vi "Select Items in Listbox_UI.vi"(8 "error in (no error)":errorcluster, 10 "Coords":T5, 11 "Input ListBox Cluster":T1) -> (0 "error out":errorcluster, 3 "ListBox Cluster out":T1)   [LabVIEW 2015, in "ZenGage v3.0 UI.lvclass"]
doc: "This VI checks for selected and unselected measurements."
uses:
  ZenGage v3.0 UI.lvclass
  <vilib>/Utility/miscctls.llb/LVPositionTypeDef.ctl
  Type Definitions/Edit tolerance settings/Edit Tolerance Input.ctl
  Type Definitions/Edit tolerance settings/ETL controls.ctl
  Type Definitions/Edit tolerance settings/Rack Selection.ctl
  <vilib>/Utility/miscctls.llb/LVPoint32TypeDef.ctl
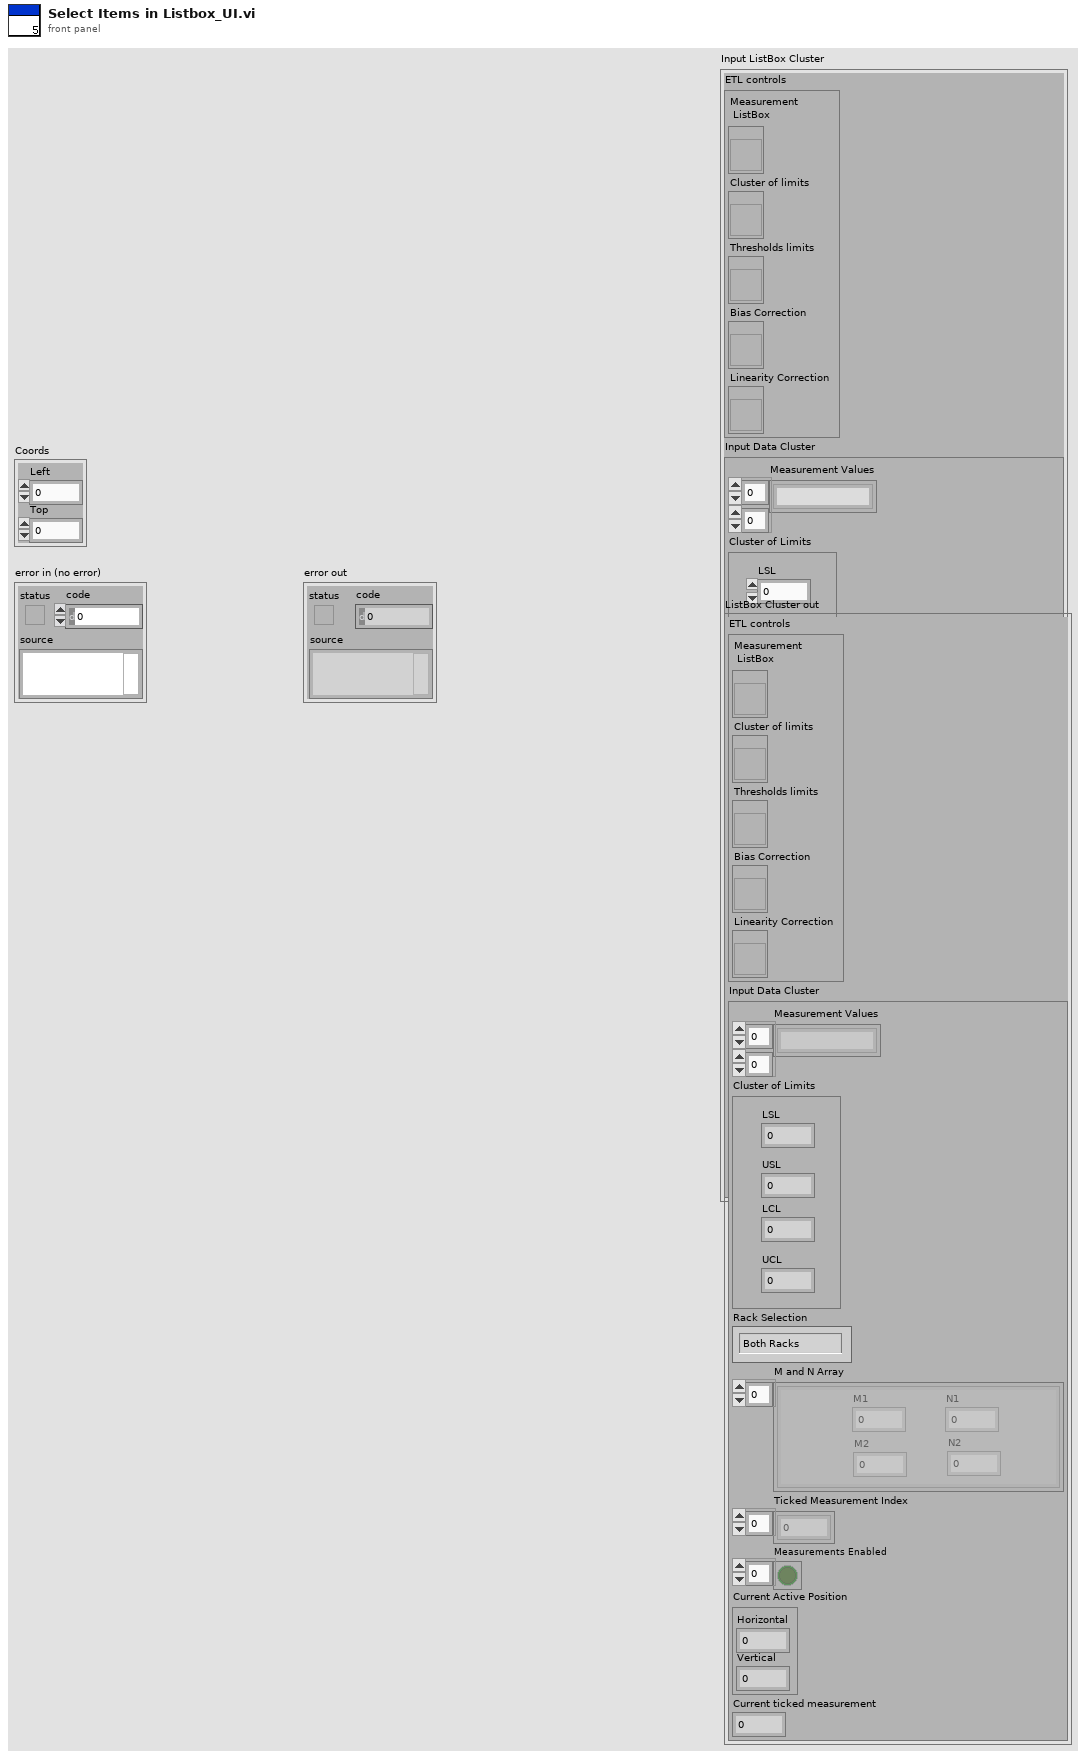
[diagram p1: front panel]
types:
  T1 = typedef "ZenGage v3.0 UI.lvclass/Edit Tolerance Input.ctl" = cluster{"ETL controls":T2, "Input Data Cluster":cluster{"Measurement Values":string[][], "Cluster of Limits":cluster{"LSL":dbl, "USL":dbl, "LCL":dbl, "UCL":dbl}, "Rack Selection":T3, "M and N Array":cluster{"M1":u64, "M2":u64, "N1":u64, "N2":u64}[], "Ticked Measurement Index":u32[], "Measurements Enabled":bool[], "Current Active Position":T4, "Current ticked measurement":dbl}}
  T2 = typedef "ETL controls.ctl" = cluster{"Measurement\n ListBox":refnum<vi>, "Cluster of limits":refnum<vi>, "Thresholds limits":refnum<vi>, "Bias Correction":refnum<vi>, "Linearity Correction":refnum<vi>}
  T3 = typedef "ZenGage v3.0 UI.lvclass/Rack Selection.ctl" = enum16{"Both Racks", "Rack 2", "Rack 1"}
  T4 = typedef "LVPoint32TypeDef.ctl" = cluster{"Horizontal":i32, "Vertical":i32}
  T5 = typedef "LVPositionTypeDef.ctl" = cluster{"Left":i32, "Top":i32}
  T6 = typedef "LVRowAndColumnTypeDef.ctl" = cluster{"Row":i32, "Column":i32}
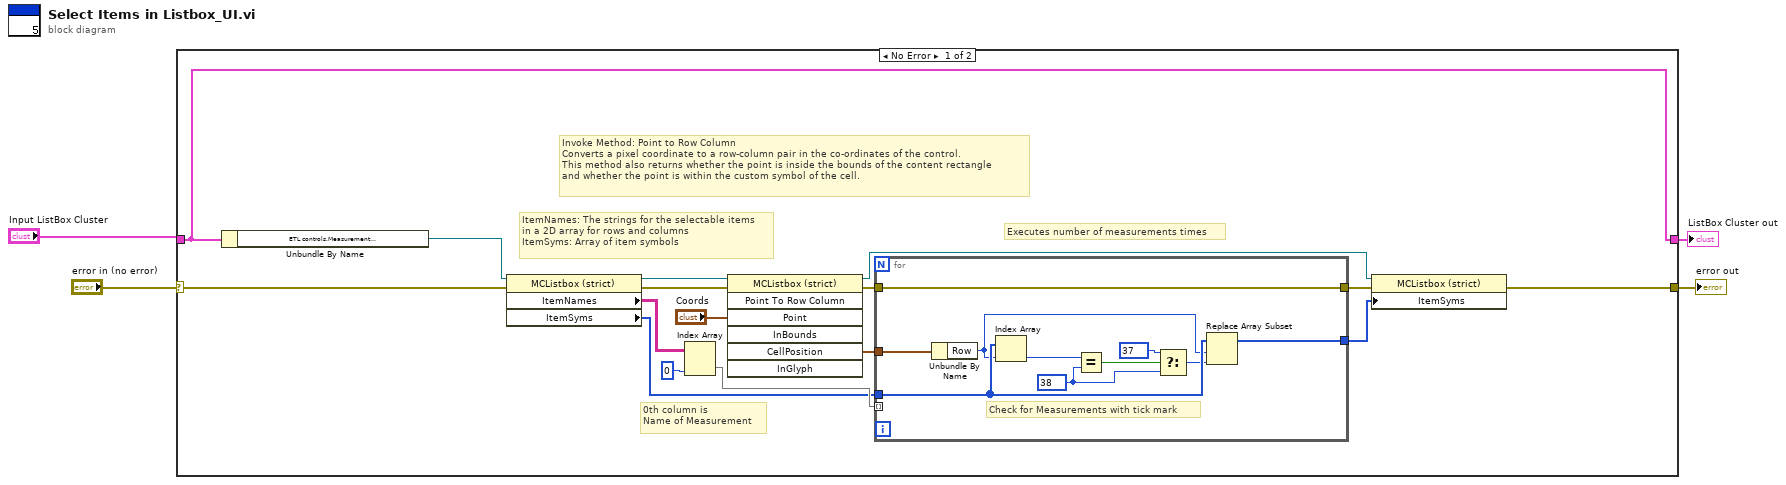
[diagram p0: block diagram]
diagram:
  n1 = case shown="No Error" "error in (no error)" {
    selector: "error in (no error)" -> [w19 w32]
    tunnel: [w18 w32] -> w3
    tunnel: [w20 w31] -> w1
    tunnel: "Input ListBox Cluster" -> [w20 w31]
    frame No Error {
      # "Executes number of measurements times"
      # "Invoke Method: Point to Row Column\nConverts a pixel coordinate to a row-column pair in the co-ordinates of the control.\nThis method also returns whether the point is inside the bounds of the content rectangle\nand whether the point is within the custom symbol of the cell."
      # "0th column is\nName of Measurement"
      # "ItemNames: The strings for the selectable items\nin a 2D array for rows and columns\nItemSyms: Array of item symbols"
      n2 = Unbundle By Name(w20) -> ("ETL controls.Measurement\n ListBox"=w5:refnum<vi>)
      n3 = property on="Property Node" class="MCListbox (strict)"(reference=w5, error in=w19) -> (reference out=w12:refnum<vi>, error out=w17:errorcluster, "ItemNames"=w7:string[][], "ItemSyms"=w6:i32[])
      n4 = Index Array(array=w7, index (col)=0 ("disabled index (col)")) -> (element=w8:string[])  [unwired: 1 in]
      n5 = invoke on="Invoke Node" class="MCListbox (strict)" method="Point To Row Column"(reference=w12, error in=w17, "Point"="Coords") -> (reference out=w11:refnum<vi>, error out=w10:errorcluster, "CellPosition"=w15:T6)  [unwired: 4 in, 4 out]
      n6 = for {
        tunnel: w15 -> [w28]
        tunnel: w8 -> [_] mode=indexing
        tunnel: w6 -> [w30]
        tunnel: [w29] -> w16
        tunnel: w10 -> [w21]
        tunnel: [w21] -> w9
        w24 = 38
        # "Check for Measurements with tick mark"
        n7 = Unbundle By Name(w28) -> ("Row"=w22:i32)
        n8 = Index Array "Index Array"(array=w30, index=w22) -> (element=w27:i32)
        n9 = Equal?(x=w27, y=w24) -> (x = y?=w26:bool)
        n10 = Select(t=37, s=w26, f=w24) -> (s? t:f=w25:i32)
        n11 = Replace Array Subset "Replace Array Subset"(array=w30, new element=w25, index=w22) -> (w29:i32[])
      }
      n12 = property on="Property Node" class="MCListbox (strict)"(reference=w11, error in=w9, "ItemSyms"=w16) -> (error out=w18:errorcluster)  [unwired: 1 out]
    }
    frame Error {
    }
  }
  "error out" <- w3
  "ListBox Cluster out" <- w1
